vi "Parameters_GetHomingParams.vi"(8 "error in (no error)":errorcluster, 11 "Parameters":dbl[](array[numeric])) -> (0 "error out":errorcluster, 3 "Reference Move Parameters":T1={"Reference Move Mode"=3, "Start Search Forward"=FALSE, "Stop on FWD Edge"=FALSE, "Approach Forward"=FALSE, "Velocity"=0.0, "Acceleration"=0.0})   [LabVIEW 2017, in "WordManipulationLibrary.lvlib"]
uses:
  WordManipulationLibrary.lvlib
  ReferenceMoveParameters.ctl
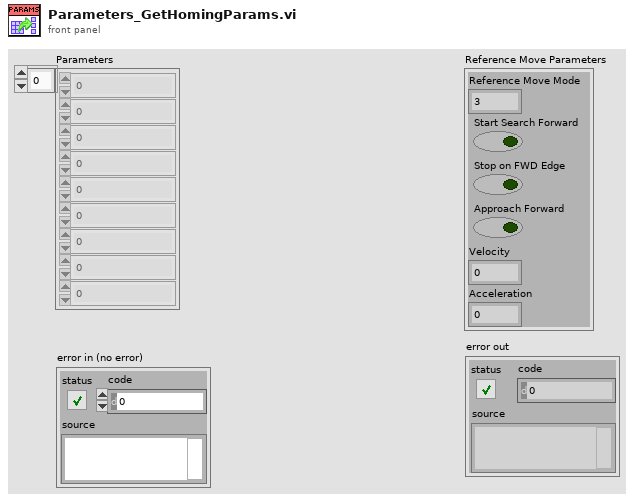
[diagram p1: front panel]
types:
  T1 = typedef "WordManipulationLibrary.lvlib/ReferenceMoveParameters.ctl" = cluster{"Reference Move Mode":i32, "Start Search Forward":bool, "Stop on FWD Edge":bool, "Approach Forward":bool, "Velocity":dbl, "Acceleration":dbl}
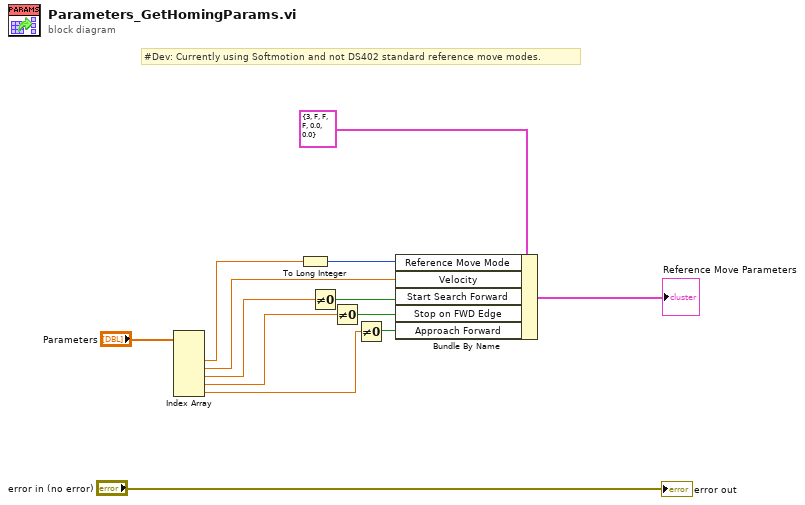
[diagram p0: block diagram]
diagram:
  # "#Dev: Currently using Softmotion and not DS402 standard reference move modes."
  n1 = Index Array(array="Parameters") -> (element #2=w10:dbl, element #3=w9:dbl, element #4=w7:dbl, element #5=w4:dbl, element #6=w3:dbl)  [unwired: 6 in, 1 out]
  n2 = To Long Integer(number=w10) -> (32bit integer=w11:i32)
  n3 = Not Equal To 0?(x=w7) -> (x != 0?=w8:bool)
  n4 = Not Equal To 0?(x=w4) -> (x != 0?=w6:bool)
  n5 = Not Equal To 0?(x=w3) -> (x != 0?=w5:bool)
  n6 = Bundle By Name(cluster=T1 {"Reference Move Mode"=3, "Start Search Forward"=FALSE, "Stop on FWD Edge"=FALSE, "Approach Forward"=FALSE, "Velocity"=0.0, "Acceleration"=0.0} ("output cluster 2"), "Reference Move Mode"=w11, "Velocity"=w9, "Start Search Forward"=w8, "Stop on FWD Edge"=w6, "Approach Forward"=w5) -> (→"Reference Move Parameters":T1)
  "error out" <- "error in (no error)"
